vi "Wrist and Intake.vi"   [LabVIEW 2018]
uses:
  Cargo Intake Cases.ctl
  Downloads/2018Robot-master/2018Robot-master/Common Code/Utilities/Change Detect.vi
  Downloads/2018Robot-master/2018Robot-master/Common Code/Utilities/Change Detect Boolean.vi
  <vilib>/Rock Robotics/Network Tables/NT Read Boolean.vi
  Robot Global Data.vi
types:
  T1 = enum16{"Home", "Hatch Push", "Hatch Out Delay", "Hatch Out"}
  T2 = typedef "Cargo Intake Cases.ctl" = enum16{"Home", "Home Button Hold", "Cargo Intake", "Cargo Intake Button Hold"}
  T3 = typedef "WPI_DigitalInputDevRef.ctl" = cluster{"DevStatus":errorcluster, "DIO Channel":T4}
  T4 = typedef "FPGA_DIOChannel.ctl" = enum8{"DIO 0", "DIO 1", "DIO 2", "DIO 3", "DIO 4", "DIO 5", "DIO 6", "DIO 7", "DIO 8", "DIO 9", "DIO MXP 0", "DIO MXP 1", "DIO MXP 2", "DIO MXP 3", "DIO MXP 4", "DIO MXP 5", "DIO MXP 6", "DIO MXP 7", "DIO MXP 8", "DIO MXP 9", "DIO MXP 10", "DIO MXP 11", "DIO MXP 12", "DIO MXP 13", "DIO MXP 14", "DIO MXP 15", "SPI Port CS1", "SPI Port CS2", "SPI Port CS3", "SPI Port MISO", "SPI Port MOSI", "Invalid"}
  T5 = enum16{"Home", "Button Hold", "Hold Pos", "Cargo release"}
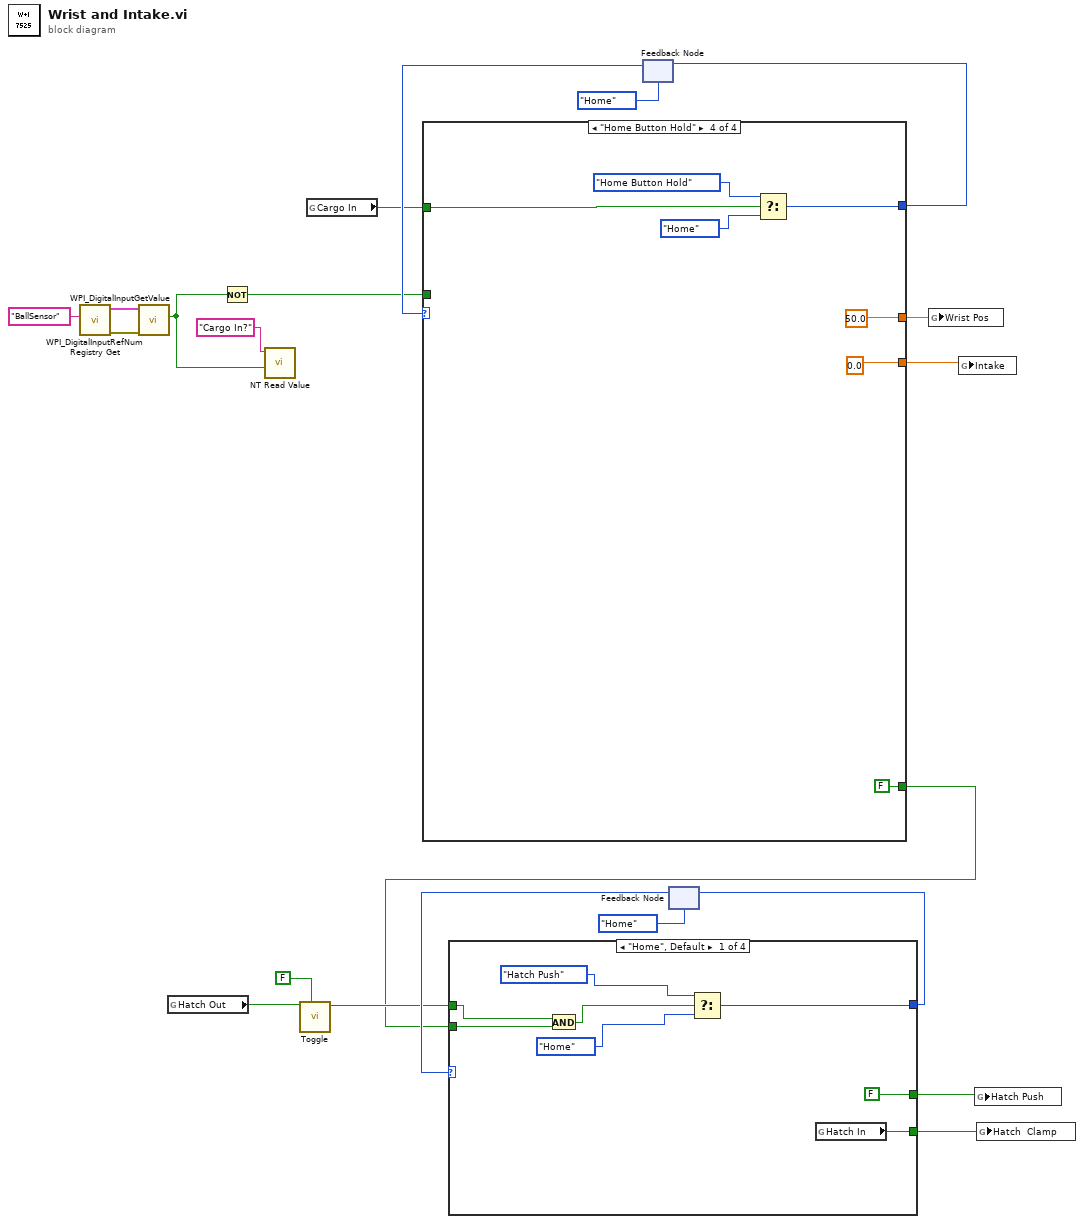
[diagram p0: block diagram]
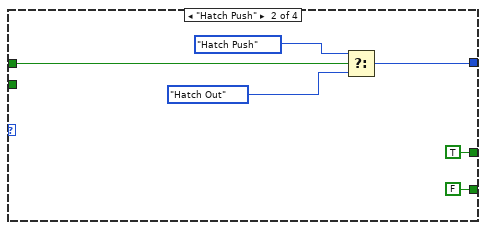
[diagram p2: hidden frame]
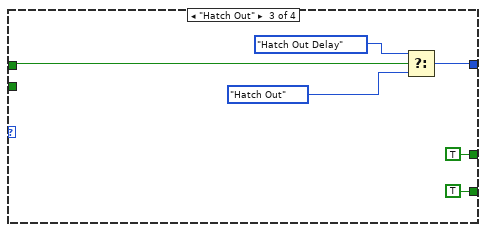
[diagram p3: hidden frame]
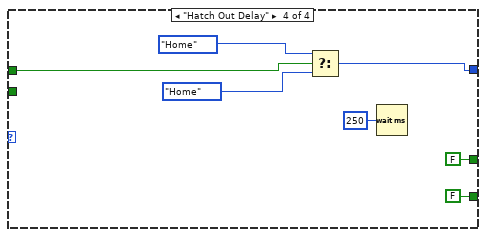
[diagram p4: hidden frame]
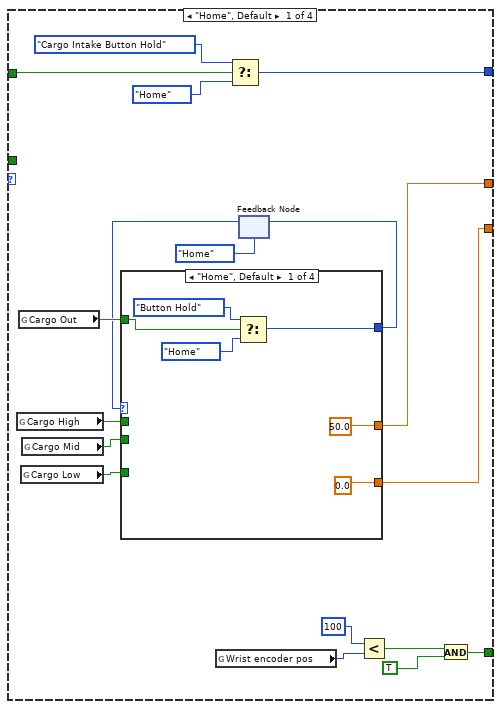
[diagram p5: hidden frame]
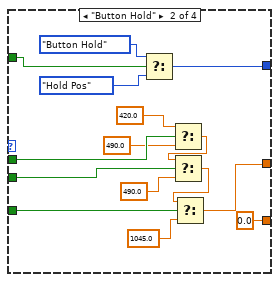
[diagram p6: hidden frame]
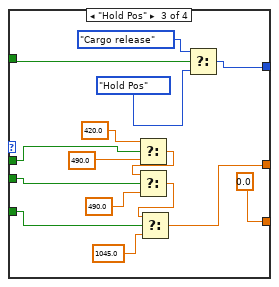
[diagram p7: hidden frame]
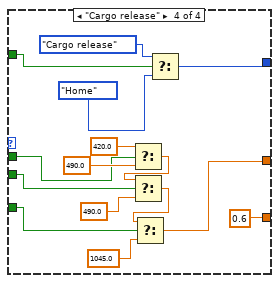
[diagram p8: hidden frame]
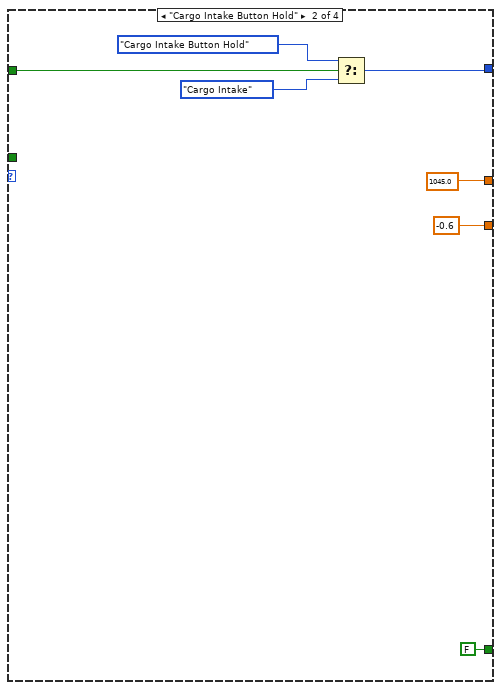
[diagram p9: hidden frame]
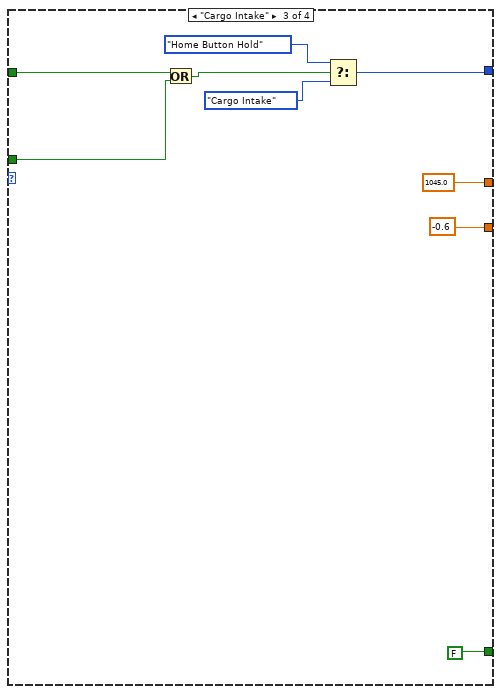
[diagram p10: hidden frame]
diagram:
  n1 = call <vilib>:"WPI_DigitalInputRefNum Registry Get.vi"("refnum name"="BallSensor") -> ("error out"=w16:errorcluster, "DigitalInputDevRef"=w17:T3)  [unwired: 9 in]
  n2 = call <vilib>:"WPI_DigitalInputGetValue.vi"("error in (no error)"=w16, "DigitalInputDevRef"=w17) -> ("Value"=w3:bool)  [unwired: 7 in, 2 out]
  n3 = global read "Robot Global Data.vi" "Hatch Out"() -> (w11:bool)
  n4 = Not(x=w3) -> (.not. x?=w1:bool)
  n5 = call-poly <vilib>:"NT Read Value.vi"("Default Value"=w3, "Name"="Cargo In?") -> ()  [unwired: 8 in, 2 out]
  n6 = call "Toggle.vi"("Initial Value"=FALSE, "In"=w11) -> ("Toggled"=w9:bool)  [unwired: 9 in]
  n7 = global read "Robot Global Data.vi" "Cargo In"() -> (w2:bool)
  n8 = feedback #1(Cargo_Intake_Cases."Home") -> (w19:T2)
  n9 = case shown="\"Home Button Hold\"" w19 {
    tunnel: [w39 w95 w101 w110] -> w20
    tunnel: w2 -> [w38 w94 w100 w111]
    tunnel: [w31 1045.0 ("Wrist Pos") 1045.0 ("Wrist Pos") 50.0 ("Wrist Pos")] -> w18
    tunnel: [w32 -0.6 -0.6 0.0] -> w14
    tunnel: [w34 FALSE FALSE FALSE] -> w8
    tunnel: w1 -> [_ _ w99 _]
    frame "Home", Default {
      n10 = global read "Robot Global Data.vi" "Cargo High"() -> (w24:bool)
      n11 = global read "Robot Global Data.vi" "Cargo Out"() -> (w30:bool)
      n12 = global read "Robot Global Data.vi" "Cargo Low"() -> (w26:bool)
      n13 = global read "Robot Global Data.vi" "Cargo Mid"() -> (w25:bool)
      n14 = global read "Robot Global Data.vi" "Wrist encoder pos"() -> (w37:i32)
      n15 = Select(t=Cargo_Intake_Cases."Cargo Intake Button Hold", s=w38, f=Cargo_Intake_Cases."Home") -> (s? t:f=w39:T2)
      n16 = feedback #2(T5."Home") -> (w28:T5)
      n17 = case shown="\"Home\", Default" w28 {
        tunnel: [0.0 0.0 0.0 0.6] -> w32
        tunnel: [50.0 ("Wrist Pos") w50 w62 w79] -> w31
        tunnel: w30 -> [w42 w56 w73 w88]
        tunnel: [w40 w57 w72 w87] -> w27
        tunnel: w26 -> [_ w54 w63 w78]
        tunnel: w25 -> [_ w51 w64 w77]
        tunnel: w24 -> [_ w49 w66 w76]
        frame "Home", Default {
          n18 = Select(t=T5."Button Hold", s=w42, f=T5."Home") -> (s? t:f=w40:T5)
        }
        frame "Button Hold" {
          n19 = Select(t=T5."Button Hold", s=w56, f=T5."Hold Pos") -> (s? t:f=w57:T5)
          n20 = Select(t=420.0, s=w49, f=490.0) -> (s? t:f=w48:dbl)
          n21 = Select(t=w48, s=w51, f=490.0) -> (s? t:f=w53:dbl)
          n22 = Select(t=w53, s=w54, f=1045.0 ("Wrist Pos")) -> (s? t:f=w50:dbl)
        }
        frame "Hold Pos" {
          n23 = Select(t=420.0, s=w66, f=490.0) -> (s? t:f=w65:dbl)
          n24 = Select(t=w65, s=w64, f=490.0) -> (s? t:f=w69:dbl)
          n25 = Select(t=w69, s=w63, f=1045.0 ("Wrist Pos")) -> (s? t:f=w62:dbl)
          n26 = Select(t=T5."Cargo release", s=w73, f=T5."Hold Pos") -> (s? t:f=w72:T5)
        }
        frame "Cargo release" {
          n27 = Select(t=420.0, s=w76, f=490.0) -> (s? t:f=w81:dbl)
          n28 = Select(t=w81, s=w77, f=490.0) -> (s? t:f=w84:dbl)
          n29 = Select(t=w84, s=w78, f=1045.0 ("Wrist Pos")) -> (s? t:f=w79:dbl)
          n30 = Select(t=T5."Cargo release", s=w88, f=T5."Home") -> (s? t:f=w87:T5)
        }
      }
      n31 = feedback-in #2(w27) -> ()
      n32 = Less?(x=100, y=w37) -> (x < y?=w33:bool)
      n33 = And(x=w33, y=TRUE) -> (x .and. y?=w34:bool)
    }
    frame "Cargo Intake Button Hold" {
      n34 = Select(t=Cargo_Intake_Cases."Cargo Intake Button Hold", s=w94, f=Cargo_Intake_Cases."Cargo Intake") -> (s? t:f=w95:T2)
    }
    frame "Cargo Intake" {
      n35 = Or(x=w100, y=w99) -> (x .or. y?=w98:bool)
      n36 = Select(t=Cargo_Intake_Cases."Home Button Hold", s=w98, f=Cargo_Intake_Cases."Cargo Intake") -> (s? t:f=w101:T2)
    }
    frame "Home Button Hold" {
      n37 = Select(t=Cargo_Intake_Cases."Home Button Hold", s=w111, f=Cargo_Intake_Cases."Home") -> (s? t:f=w110:T2)
    }
  }
  n38 = feedback-in #1(w20) -> ()
  n39 = feedback #3(T1."Home") -> (w12:T1)
  n40 = case shown="\"Home\", Default" w12 {
    tunnel: [w121 w124 w130 w138] -> w7
    tunnel: w9 -> [w120 w127 w131 w137]
    tunnel: w8 -> [w118 _ _ _]
    tunnel: [FALSE TRUE TRUE FALSE] -> w6
    tunnel: [w114 FALSE ("Hatch In") TRUE ("Hatch In") FALSE ("Hatch In")] -> w5
    frame "Home", Default {
      n41 = And(x=w120, y=w118) -> (x .and. y?=w119:bool)
      n42 = Select(t=T1."Hatch Push", s=w119, f=T1."Home") -> (s? t:f=w121:T1)
      n43 = global read "Robot Global Data.vi" "Hatch In"() -> (w114:bool)
    }
    frame "Hatch Push" {
      n44 = Select(t=T1."Hatch Push", s=w127, f=T1."Hatch Out") -> (s? t:f=w124:T1)
    }
    frame "Hatch Out" {
      n45 = Select(t=T1."Hatch Out Delay", s=w131, f=T1."Hatch Out") -> (s? t:f=w130:T1)
    }
    frame "Hatch Out Delay" {
      n46 = Select(t=T1."Home", s=w137, f=T1."Home") -> (s? t:f=w138:T1)
      n47 = Wait (ms)(milliseconds to wait=u32 250) -> ()  [unwired: 1 out]
    }
  }
  n48 = feedback-in #3(w7) -> ()
  n49 = global write "Robot Global Data.vi" "Wrist Pos"(w18) -> ()
  n50 = global write "Robot Global Data.vi" "Intake"(w14) -> ()
  n51 = global write "Robot Global Data.vi" "Hatch Push"(w6) -> ()
  n52 = global write "Robot Global Data.vi" "Hatch  Clamp"(w5) -> ()
